vi "DSF.Engine.Framework.Initialize.Transfer Groups.vi"(8 "error in (no error)":errorcluster, 10 "All Transfers":refnum<class "DSF.Engine.Transfer.lvclass">[](array[class]), 11 "Framework in":refnum<class "DSF.Engine.Framework.lvclass">) -> (0 "error out":errorcluster, 2 "All Transfer Groups":refnum<class "DSF.Engine.Transfer Group.lvclass">[](array[class]), 3 "Framework out":refnum<class "DSF.Engine.Framework.lvclass">)   [LabVIEW 2017, in "DSF.Engine.lvlib" / "DSF.Engine.Framework.lvclass"]
uses:
  DSF.Engine.Framework.lvclass
  Transfer/DSF.Engine.Transfer Group.lvclass
  Transfer/DSF.Engine.Transfer.lvclass
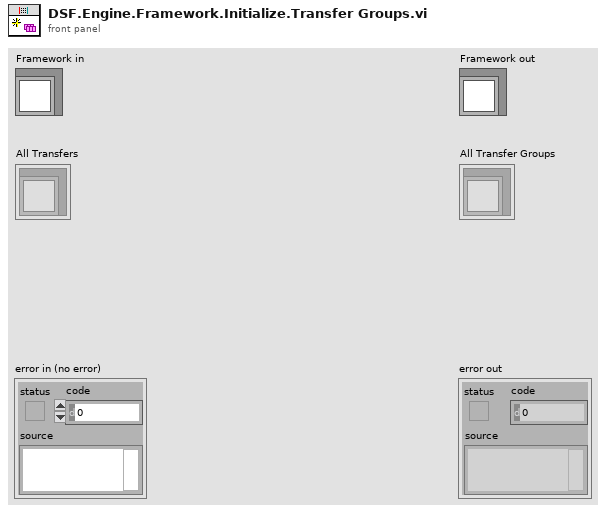
[diagram p1: front panel]
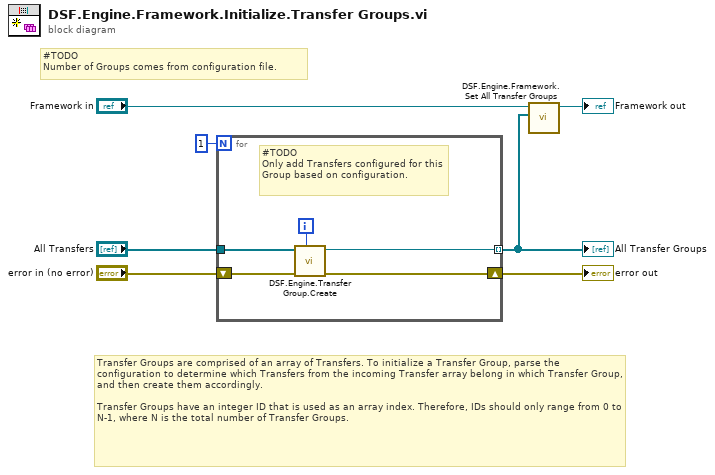
[diagram p0: block diagram]
diagram:
  # "#TODO\nNumber of Groups comes from configuration file."
  # "Transfer Groups are comprised of an array of Transfers. To initialize a Transfer Group, parse the configuration to determine which Transfers from the incoming Transfer array belong in which Transfer Group, and then create them accordingly.\n\nTransfer Groups have an integer ID that is used as an array index. Therefore, IDs should only range from 0 to N-1, where N is the total number of Transfer Groups."
  n1 = for {
    N: 1 -> [_]
    tunnel: "All Transfers" -> [w11]
    shift-right: [w12] -> w4
    shift-left: "error in (no error)" -> [w10]
    tunnel: [w9] -> w1 mode=indexing
    i -> [w8]
    # "#TODO\nOnly add Transfers configured for this Group based on configuration."
    n2 = call "DSF.Engine.Transfer Group.Create.vi"("id"=w8, "error in (no error)"=w10, "Transfers"=w11) -> ("error out"=w12:errorcluster, "Transfer Group out"=w9:refnum<class "DSF.Engine.Transfer Group.lvclass">)  [unwired: 7 in]
  }
  "error out" <- w4
  "All Transfer Groups" <- w1
  n3 = call "DSF.Engine.Framework.Set All Transfer Groups.vi"("All Transfer Groups"=w1, "Framework in"="Framework in") -> ("Framework out"=→"Framework out":refnum<class "DSF.Engine.Framework.lvclass">)  [unwired: 9 in]
